vi "ENA_Configure Trigger.vi"(7 "Trigger Type":enum16{"Internal", "Manual", "External"}(ring), 8 "error in (no error)":errorcluster, 11 "VISA resource name":refnum<visa-resource-name>) -> (0 "error out":errorcluster, 3 "VISA resource name out":refnum<visa-resource-name>)   [LabVIEW 2013]
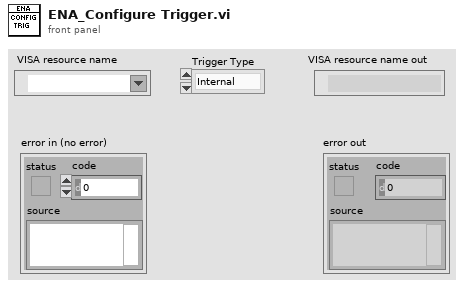
[diagram p1: front panel]
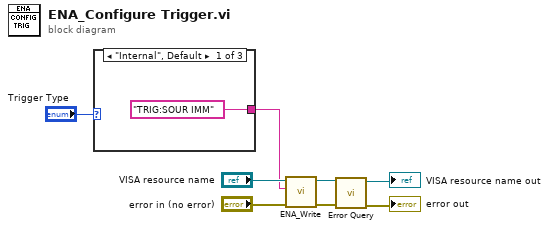
[diagram p0: block diagram]
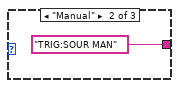
[diagram p2: hidden frame]
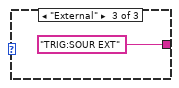
[diagram p3: hidden frame]
diagram:
  n1 = case shown="\"Internal\", Default" "Trigger Type" {
    tunnel: ["TRIG:SOUR IMM" "TRIG:SOUR MAN" "TRIG:SOUR EXT"] -> w1
    frame "Internal", Default {
    }
    frame "Manual" {
    }
    frame "External" {
    }
  }
  n2 = call "ENA_Write.vi"("error in (no error)"="error in (no error)", "String ()"=w1, "VISA resource name"="VISA resource name") -> ("error out"=w5:errorcluster, "VISA resource name out"=w6:refnum<visa-resource-name>)  [unwired: 6 in, 1 out]
  n3 = call "Error Query.vi"("error in (no error)"=w5, "VISA resource name"=w6) -> ("error out"=→"error out":errorcluster, "VISA resource name out"=→"VISA resource name out":refnum<visa-resource-name>)  [unwired: 6 in, 2 out]
